vi "RSZVB Marker Search Range.vi"(5 "Search Range (0: Full Span)":i32(ring) items=["Full Span", "Range 1", "Range 2", "Range 3", "Range 4", "Range 5", "Range 6", "Range 7", "Range 8", "Range 9", "Range 10"], 6 "Stop (0.0)":dbl format="%^.3e", 7 "Start (0.0)":dbl format="%^.3e", 8 "error in (no error)":errorcluster {"code" format="%.0x"}, 9 "Marker (1)":i32=1, 10 "Channel (Trace) (1)":i32=1, 11 "VISA session":refnum<visa-resource-name>) -> (0 "error out":errorcluster {"code" format="%.0x"}, 3 "dup VISA session":refnum<visa-resource-name>)   [LabVIEW 2011]
doc: "This VI defines search ranges for the maximum/minimum or target search. Assigns a search range to marker and define the start and stop values.\n\nRemote-control command(s):\nCALCulate<Ch/Tr>:MARKer<Mk>:FUNCtion:DOMain:USER <numeric_value>\nCALCulate<Ch/Tr>:MARKer<Mk>:FUNCtion:DOMain:USER:STARt <numeric_value>\nCALCulate<Ch/Tr>:MARKer<Mk>:FUNCtion:DOMain:USER:STOP <numeric_value>"
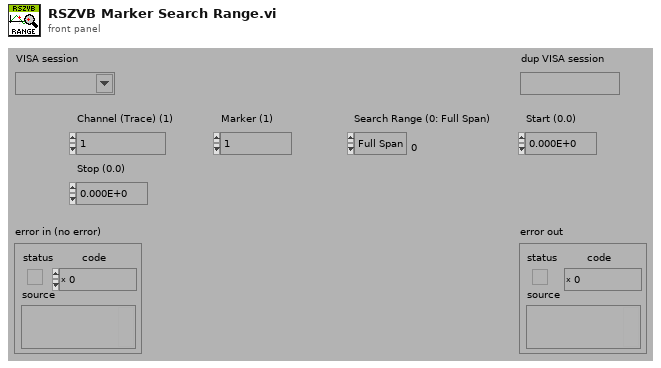
[diagram p1: front panel]
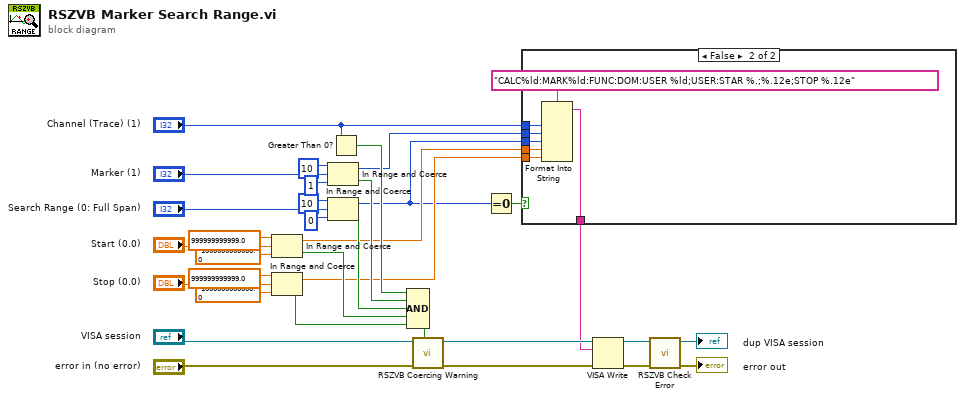
[diagram p0: block diagram]
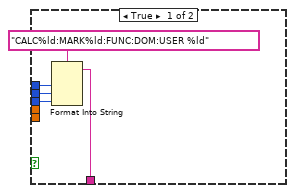
[diagram p2: hidden frame]
diagram:
  n1 = In Range and Coerce(upper limit=999999999999.0, x="Start (0.0)", lower limit=-1000000000000.0 ("upper limit")) -> (coerced(x)=w4:dbl, In Range?=w7:bool)
  n2 = In Range and Coerce(upper limit=999999999999.0, x="Stop (0.0)", lower limit=-1000000000000.0 ("upper limit")) -> (coerced(x)=w3:dbl, In Range?=w8:bool)
  n3 = In Range and Coerce(upper limit=10, x="Marker (1)", lower limit=1) -> (coerced(x)=w6:i32, In Range?=w26:bool)
  n4 = In Range and Coerce(upper limit=10, x="Search Range (0: Full Span)", lower limit=0) -> (coerced(x)=w1:i32, In Range?=w21:bool)
  n5 = Greater Than 0?(x="Channel (Trace) (1)") -> (x > 0?=w29:bool)
  n6 = Compound Arithmetic op=AND(w29, w26, w21, w7, w8) -> (w23:bool)
  n7 = call "RSZVB Coercing Warning.vi"("In Range?"=w23, "error in (no error)"="error in (no error)", "VISA session"="VISA session") -> ("error out"=w32:errorcluster, "dup VISA session"=w33:refnum<visa-resource-name>)  [unwired: 7 in]
  n8 = Equal To 0?(x=w1) -> (x = 0?=w2:bool)
  n9 = case shown="False" w2 {
    tunnel: [w37 w44] -> w22
    tunnel: w1 -> [w36 w43]
    tunnel: w6 -> [w35 w42]
    tunnel: "Channel (Trace) (1)" -> [w34 w41]
    tunnel: w4 -> [_ w40]
    tunnel: w3 -> [_ w39]
    frame True {
      n10 = Format Into String(format string="CALC%ld:MARK%ld:FUNC:DOM:USER %ld", w34, w35, w36) -> (resulting string=w37:string)  [unwired: 2 in, 1 out]
    }
    frame False {
      n11 = Format Into String(format string="CALC%ld:MARK%ld:FUNC:DOM:USER %ld;USER:STAR %.;%.12e;STOP %.12e", w41, w42, w43, w40, w39) -> (resulting string=w44:string)  [unwired: 2 in, 1 out]
    }
  }
  n12 = VISA Write(VISA resource name=w33, write buffer=w22, error in (no error)=w32) -> (VISA resource name out=w30:refnum<visa-resource-name>, error out=w31:errorcluster)  [unwired: 1 out]
  n13 = call "RSZVB Check Error.vi"("error in (no error)"=w31, "VISA session"=w30) -> ("error out"=→"error out":errorcluster, "dup VISA session"=→"dup VISA session":refnum<visa-resource-name>)  [unwired: 8 in]
